vi "Setedge.vi"(8 "error in (no error)":errorcluster, 10 "Set_Val":T1, 11 "OneOfTemplate in":refnum<class "nidaqmx_grpc_CreateCIFreqChanRequest_edge_enum.lvclass">) -> (0 "error out":errorcluster, 3 "OneOfTemplate out":refnum<class "nidaqmx_grpc_CreateCIFreqChanRequest_edge_enum.lvclass">)   [LabVIEW 2021, in "NI DAQmx_server.lvlib" / "nidaqmx_grpc_CreateCIFreqChanRequest_edge_enum.lvclass"]
uses:
  nidaqmx_grpc_CreateCIFreqChanRequest_edge_enum.lvclass
  nidaqmx_grpc_Edge1.ctl
  nidaqmx_grpc_CreateCIFreqChanRequest_edge_enum.lvclass/nidaqmx_grpc_CreateCIFreqChanRequest_edge_enum.ctl
  NI DAQmx_server.lvlib
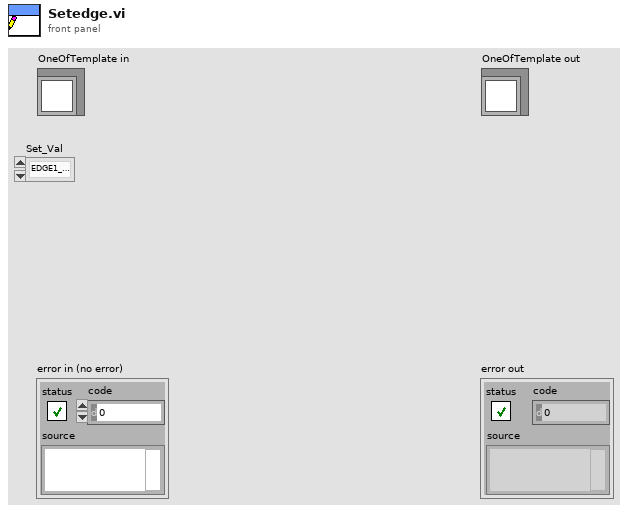
[diagram p1: front panel]
types:
  T1 = typedef "NI DAQmx_server.lvlib/nidaqmx_grpc_Edge1.ctl" = enum32{"EDGE1_UNSPECIFIED", "EDGE1_RISING", "EDGE1_FALLING"}
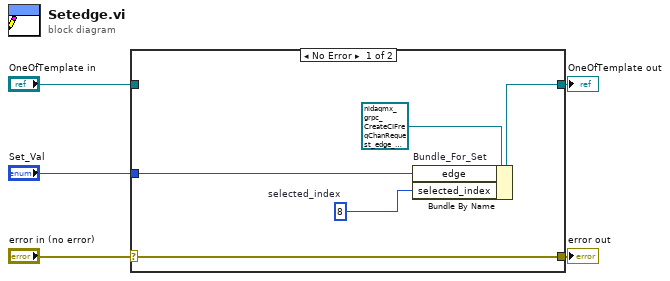
[diagram p0: block diagram]
diagram:
  n1 = case shown="No Error" "error in (no error)" {
    selector: "error in (no error)" -> [w10 w11]
    tunnel: [w10 w11] -> w4
    tunnel: [w9 w12] -> w2
    tunnel: "OneOfTemplate in" -> [_ w12]
    tunnel: "Set_Val" -> [w8 _]
    frame No Error {
      w7 = 8  # selected_index
      n2 = Bundle By Name "Bundle_For_Set"(cluster=refnum<class "nidaqmx_grpc_CreateCIFreqChanRequest_edge_enum.lvclass"> refnum ("OneOfTemplate in"), "edge"=w8, "selected_index"=w7) -> (w9:refnum<class "nidaqmx_grpc_CreateCIFreqChanRequest_edge_enum.lvclass">)
    }
    frame Error {
    }
  }
  "error out" <- w4
  "OneOfTemplate out" <- w2
